vi "Initialize Comm.vi"(0 "Device ID":T1(ring), 7 "immer erster aufruf?":bool, 11 "error in":errorcluster) -> (4 "Device ID Out":T1(ring), 15 "error out":errorcluster)   [LabVIEW 2010]
doc: "This VI initializes communication between your computer and the Robo Interface. It cleans up any communication threads still open from a previous run."
uses:
  Robo Interface.dll
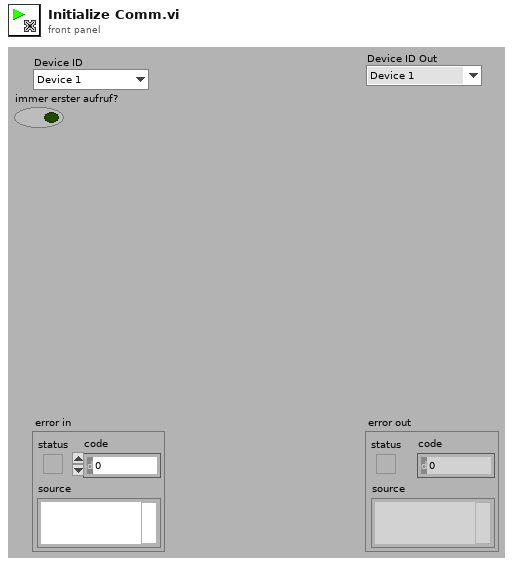
[diagram p1: front panel]
types:
  T1 = enum16{"Device 1", "Device 2", "Device 3", "Device 4", "Device 5", "Device 6", "Device 7", "Device 8"}
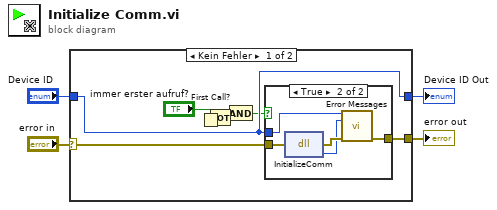
[diagram p0: block diagram]
diagram:
  n1 = case shown="Kein Fehler" "error in" {
    selector: "error in" -> [w11 w19]
    tunnel: [w10 w19] -> w3
    tunnel: "Device ID" -> [w9 w18]
    tunnel: [w9 w18] -> w1
    frame No Error {
      n2 = First Call?() -> (First Call?: T/F=w8:bool)
      n3 = Not(x=w8) -> (.not. x?=w5:bool)
      n4 = And(x="immer erster aufruf?", y=w5) -> (x .and. y?=w7:bool)
      n5 = case shown="TRUE" w7 {
        tunnel: w11 -> [w12 w17]
        tunnel: [w12 w15] -> w10
        tunnel: w9 -> [_ w13]
        frame False {
        }
        frame True {
          n6 = dll-call lib="D:/Aron/LabVIEW-Programmierung/a.F.b.u.s.A/robo_interface_distribute/Robo Interface/Advanced/Robo Interface.dll" fn="InitializeComm"(error in=w17) -> (error out=w16:errorcluster, "return type"=w14:i32)  [unwired: 2 in, 1 out]
          n7 = call "Error Messages.vi"("Device ID"=w13, "Error Code"=w14, "error in (no error)"=w16) -> ("error out"=w15:errorcluster)  [unwired: 12 out]
        }
      }
    }
    frame Error {
    }
  }
  "error out" <- w3
  "Device ID Out" <- w1
